vi "Receive Boolean Value Msg.vi"(8 "error in (no error)":errorcluster, 10 "BooleanValueMsg":refnum<class "BooleanValueMsg.lvclass">, 11 "TwoButtonDialogBox in":refnum<class "TwoButtonDialogBox.lvclass">) -> (0 "error out":errorcluster, 3 "TwoButtonDialogBox out":refnum<class "TwoButtonDialogBox.lvclass">)   [LabVIEW 2015, in "TwoButtonDialogBox.lvlib" / "TwoButtonDialogBox.lvclass"]
uses:
  TwoButtonDialogBox.lvclass
  AutoRegistration/ActorAutoRegistration Messages/BooleanValueMsg/BooleanValueMsg.lvclass
  <vilib>/ActorFramework/Actor/Actor.lvclass/Actor.ctl
  <vilib>/ActorFramework/Message Enqueuer/Message Enqueuer.lvclass/Message Enqueuer.ctl
  TwoButtonDialogBox.lvclass/TwoButtonDialogBox.ctl
  <vilib>/ActorFramework/Message Enqueuer/Init from Existing Queue.vi
  <vilib>/ActorFramework/Message Enqueuer/Enqueue.vi
  <vilib>/ActorFramework/Message Priority Queue/Priority Enqueue.vi
  <vilib>/ActorFramework/Message Enqueuer/Message Enqueuer.lvclass
  IDialogBox/IDialogBox Abstract Messages/Abstract Dialog Return Msg/Abstract Dialog Return Msg.lvclass
  <vilib>/ActorFramework/Stop Msg/Stop Msg.lvclass
  <vilib>/ActorFramework/Actor/Actor.lvclass
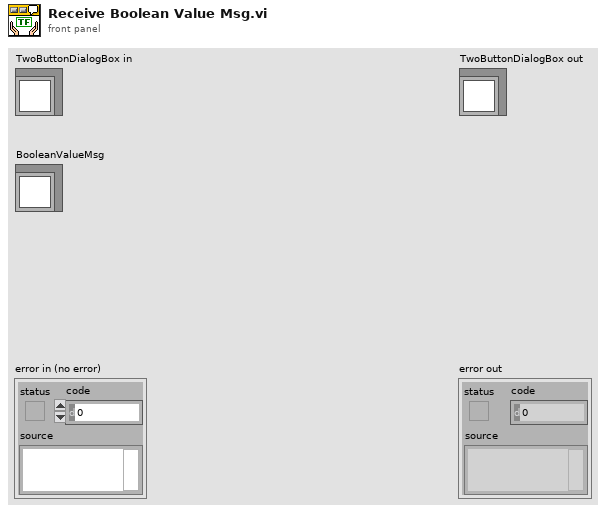
[diagram p1: front panel]
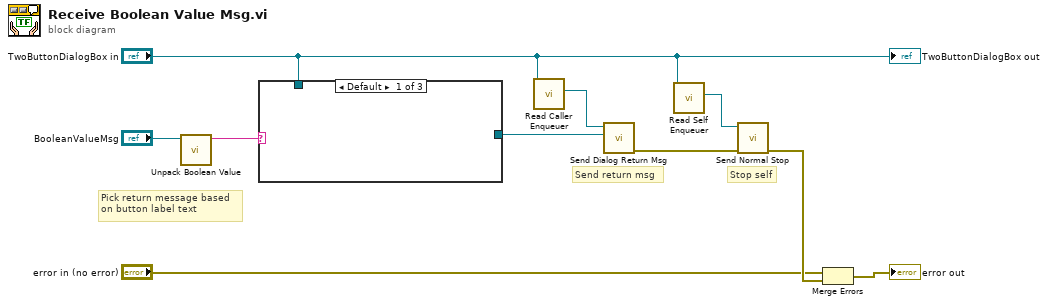
[diagram p0: block diagram]
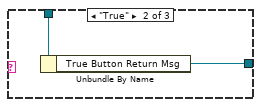
[diagram p2: hidden frame]
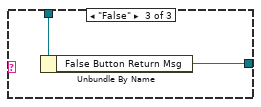
[diagram p3: hidden frame]
diagram:
  # "Pick return message based\non button label text"
  # "Stop self"
  # "Send return msg"
  n1 = call-dynamic "Unpack Boolean Value.vi"("BooleanValueMsg in"="BooleanValueMsg") -> ("Name"=w3:string)  [unwired: 9 in, 1 out]
  n2 = case shown="Default" w3 {
    tunnel: [_ w12 w14] -> w10
    tunnel: "TwoButtonDialogBox in" -> [_ w11 w13]
    frame Default {
    }
    frame "True" {
      n3 = Unbundle By Name(w11) -> ("True Button Return Msg"=w12:refnum<class "Abstract Dialog Return Msg.lvclass">)
    }
    frame "False" {
      n4 = Unbundle By Name(w13) -> ("False Button Return Msg"=w14:refnum<class "Abstract Dialog Return Msg.lvclass">)
    }
  }
  n5 = call <vilib>:"Read Caller Enqueuer.vi"("Actor"="TwoButtonDialogBox in") -> ("Caller Enqueuer"=w9:refnum<class "Message Enqueuer.lvclass">)  [unwired: 10 in]
  n6 = call "Send Dialog Return Msg.vi"("Dialog Return Msg"=w10, "Message Enqueuer in"=w9) -> ("error out"=w7:errorcluster)  [unwired: 9 in]
  n7 = call <vilib>:"Read Self Enqueuer.vi"("Actor"="TwoButtonDialogBox in") -> ("Self Enqueuer"=w8:refnum<class "Message Enqueuer.lvclass">)  [unwired: 10 in]
  n8 = call <vilib>:"Send Normal Stop.vi"("error in (no error)"=w7, "Message Enqueuer"=w8) -> ("error out"=w6:errorcluster)  [unwired: 9 in]
  n9 = Merge Errors("error in (no error)", w6) -> (→"error out":errorcluster)
  "TwoButtonDialogBox out" <- "TwoButtonDialogBox in"
